vi "Basic Qs.vi"() -> ()   [LabVIEW 2021, in "Q Async.lvlib"]
uses:
  Q Async.lvlib
panel:
  in  "Numeric":i32=3
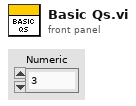
[diagram p1: front panel]
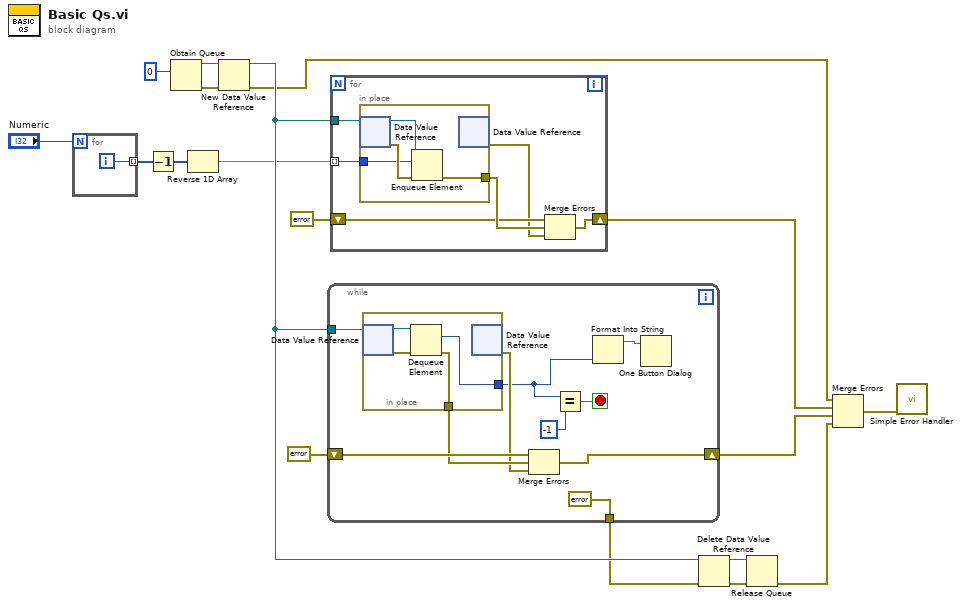
[diagram p0: block diagram]
diagram:
  n1 = for {
    N: "Numeric" -> [_]
    tunnel: [w19] -> w17 mode=indexing
    i -> [w19]
  }
  n2 = Decrement(x=w17) -> (x-1=w18:i32[])
  n3 = Obtain Queue(element data type=0) -> (queue out=w15:refnum<queue>, error out=w8:errorcluster)  [unwired: 4 in, 1 out]
  n4 = Reverse 1D Array(array=w18) -> (reversed array=w12:i32[])
  n5 = New Data Value Reference(data value=w15, error in=w8) -> (data value reference=w13:refnum<data-value>, error out=w1:errorcluster)
  n6 = while {
    tunnel: w13 -> [w27]
    tunnel: [errorcluster {"status"=FALSE, "code"=0, "source"=""} ("error in (no error)")] -> w11
    shift-right: [w23] -> w4
    shift-left: errorcluster {"status"=FALSE, "code"=0, "source"=""} ("error IO") -> [w25]
    stop <- w29 stop-if-true
    n7 = in-place {
      in-place-border: [w33] -> w20
      in-place-border: [w30] -> w24
      n8 = in-place-dvr #1(w27) -> (w32:refnum<queue>, w31:errorcluster)
      n9 = Dequeue Element(queue=w32, error in (no error)=w31) -> (element=w33:i32, error out=w30:errorcluster)  [unwired: 1 in, 2 out]
      n10 = in-place-dvr #1() -> (w22:errorcluster)  [unwired: 1 in, 1 out]
    }
    n11 = Merge Errors(w25, w24, w22) -> (w23:errorcluster)
    n12 = Equal?(x=w20, y=-1) -> (x = y?=w29:bool)
    n13 = Format Into String(w20) -> (resulting string=w21:string)  [unwired: 3 in, 1 out]
    n14 = One Button Dialog(message=w21) -> ()  [unwired: 1 in, 1 out]
  }
  n15 = for {
    tunnel: w13 -> [w39]
    tunnel: w12 -> [w38] mode=indexing
    shift-right: [w36] -> w5
    shift-left: errorcluster {"status"=FALSE, "code"=0, "source"=""} ("error out") -> [w35]
    n16 = in-place {
      in-place-border: w38 -> [w40]
      in-place-border: [w41] -> w37
      n17 = in-place-dvr #2(w39) -> (w43:refnum<queue>, w42:errorcluster)
      n18 = Enqueue Element(queue=w43, element=w40, error in (no error)=w42) -> (error out=w41:errorcluster)  [unwired: 1 in, 2 out]
      n19 = in-place-dvr #2() -> (w34:errorcluster)  [unwired: 1 in, 1 out]
    }
    n20 = Merge Errors(w35, w37, w34) -> (w36:errorcluster)
  }
  n21 = Delete Data Value Reference(data value reference=w13, error in=w11) -> (data value=w10:refnum<queue>, error out=w9:errorcluster)
  n22 = Release Queue(queue=w10, error in (no error)=w9) -> (error out=w3:errorcluster)  [unwired: 1 in, 2 out]
  n23 = Merge Errors(w1, w5, w4, w3) -> (w2:errorcluster)
  n24 = call <vilib>:"Simple Error Handler.vi"("error in (no error)"=w2) -> ()  [unwired: 4 in, 5 out]
